vi "AudioTest.Discrete Swept-Sine Measurements (Finite).vi"() -> ()   [LabVIEW 2018]
doc: "Overview:\nThis VI demonstrates simultaneous frequency response, level, and distortion measurements using a discrete swept-sine technique. This example implements analog input and analog output with 'Finite Samples' sample mode which minimizes sensitivity to bandwidth issues that can cause run-time errors when performing continuous measurements. This VI also demonstrates how finite acquisitions can be read in a single large block or in a series of smaller reads.\n\nRequirements:\nLabVIEW Full Development System\nSound and Vibration Toolkit\n\nInstructions:\n1. Connect the DUT to the DSA device.\n2. Select the AO excitation channel, AI stimulus channel, and AI response channel.\n3. Run the VI.\n\nDetails:\nThis VI performs a swept sine measurement to obtain the root-mean-square (RMS) levels of the acquired stimulus and response, the frequency response of the device under test (DUT), and the harmonic distortion on the response channel. You specify the source and measurement parameters, and the swept sine VIs handle all the DAQ-specific controls required to perform the measurement. You have direct control over the source, input, averaging, and display parameters. You also specify the engineering units to use for the swept sine measurements.\n\nYou can view the time records of the acquired stimulus and response signals. From these graphs, you can see that the transition to the next test frequency always occurs at a zero crossing to minimize non-linear disturbances to the DUT. The RMS levels, frequency response, and harmonic distortion are shown on different tabs."
uses:
  <vilib>/sound2/lvsound2.llb/Sampling Mode.ctl
  <vilib>/sound2/lvsound2.llb/Sound Data Format.ctl
  <vilib>/Utility/error.llb/DialogType.ctl
  <vilib>/addons/_NISVFA/_Generation/Signal Generation/SV Signal/SV Signal.lvclass/SV Signal.ctl
  <vilib>/addons/_NISVFA/_Generation/Signal Generation/SV Discrete Sweep/SV Discrete Sweep.lvclass/SV Discrete Sweep.ctl
  <vilib>/addons/Sound and Vibration/svt_Level/SVL AC & DC Level (Time) (1 Ch).vi
  <vilib>/addons/_NISVFA/_Shared subVIs/Common/SV Append Data (N Ch) (DBL).vi
  <vilib>/addons/_NISVFA/_Generation/Signal Generation/SV Signal/Write Leading Synchronization Pulse Enable.vi
  <vilib>/addons/_NISVFA/_Generation/Signal Generation/SV Discrete Sweep/Read All Frequencies and Amplitudes.vi
  <vilib>/addons/_NISVFA/_Generation/Signal Generation/SV Discrete Sweep/Write All Frequencies and Amplitudes.vi
  <vilib>/addons/_NISVFA/_Shared subVIs/Common/svc_Get SV Channel Info.vi
  <vilib>/Analysis/baseanly.llb/Mean.vi
  <vilib>/Analysis/baseanly.llb/Mean (DBL).vi
  <vilib>/addons/_NISVFA/_Shared subVIs/Windowing/svfa_Scaled Time Domain Window (Array).vi
  <vilib>/addons/_NISVFA/_Generation/Signal Generation/SV Discrete Sweep/Read Frequencies and Amplitudes.vi
  <vilib>/Analysis/4window.llb/Force Window.vi
  <vilib>/Analysis/4window.llb/Force Window (DBL).vi
  <vilib>/Analysis/4window.llb/Exponential Window.vi
  <vilib>/Analysis/4window.llb/Exponential Window (DBL).vi
  <vilib>/addons/_NISVFA/_Generation/Signal Generation/SV Discrete Sweep/SV Discrete Sweep.lvclass
  C:/Program Files (x86)/National Instruments/LabVIEW 2018/vi.lib/addons/_NISVFA/_Generation/Signal Generation/SV Signal/SV Signal.lvclass
  C:/Program Files (x86)/National Instruments/LabVIEW 2018/vi.lib/addons/_NISVFA/_Generation/Signal Generation/SV Function/SV Function.lvclass
  <vilib>/addons/_NISVFA/_Generation/Signal Generation/SV Discrete Sweep/Configure Frequency Sweep at Constant Amplitude.vi
  <vilib>/addons/_NISVFA/_Generation/Signal Generation/SV Signal/Write Ramp Parameters.vi
  <vilib>/addons/_NISVFA/_Generation/Signal Generation/SV Signal/Write DC Offset.vi
  <vilib>/addons/_NISVFA/_Generation/Signal Generation/SV Signal/Write Measurement Duration.vi
  <vilib>/addons/_NISVFA/_Generation/Signal Generation/SV Function/Write Measurement Cycles.vi
  <vilib>/addons/_NISVFA/_Generation/Signal Generation/SV Signal/Write Pre-Measurement Settling Duration.vi
  <vilib>/addons/_NISVFA/_Generation/Signal Generation/SV Function/Write Pre-Measurement Settling Cycles.vi
  <vilib>/addons/_NISVFA/_Generation/Signal Generation/SV Signal/Write Sample Rate.vi
  <vilib>/sound2/lvsound2.llb/Sound Output Set Volume (Single).vi
  <vilib>/sound2/lvsound2.llb/Sound Output Write (DBL Single).vi
  <vilib>/sound2/lvsound2.llb/Sound Input Read (DBL).vi
  <vilib>/addons/_NISVFA/_Shared subVIs/Data Objects/Waveforms (DBL)/SV Read Next Measurement Data.vi
  <vilib>/addons/_NISVFA/_Shared subVIs/Common/svc_Get Window Info.vi
  <vilib>/addons/_NISVFA/_Shared subVIs/Common/svc_Unit Label to Engineering Units.vi
  <vilib>/addons/_NISVFA/_Shared subVIs/Common/svc_Engineering Units to Unit Label.vi
  <vilib>/addons/_NISVFA/_Spectrum Processing/subVIs/svfa_Spectrum Info Window to windowTd Type Def.vi
  <vilib>/Analysis/0measdsp.llb/Scaled Time Domain Window.vi
  <vilib>/Analysis/0measdsp.llb/Scaled Time Domain Window (DBL).vi
  <vilib>/Utility/error.llb/Error Cluster From Error Code.vi
  <vilib>/Analysis/baseanly.llb/Std Deviation and Variance.vi
  <vilib>/addons/_NISVFA/_Shared subVIs/Common/svc_Caller VI Returned in Error Source.vi
  <vilib>/addons/Sound and Vibration/svt_Single Tone Measurements/SVT Gain and Phase (Time).vi
  <vilib>/addons/Sound and Vibration/svt_Distortion/SVT THD and Harmonic Components (Frequency) (1 Ch).vi
  <vilib>/addons/_NISVFA/_Generation/Signal Generation/SV Signal/SV Signal.lvclass
  <vilib>/addons/_NISVFA/_Shared subVIs/Data Objects/Waveforms (DBL)/Waveforms (N Ch).lvclass
  <vilib>/addons/Sound and Vibration/svt_Distortion/SoundVib_Distortion.lvlib
  <vilib>/addons/Sound and Vibration/svt_Single Tone Measurements/SoundVib_SingleTone.lvlib
  Program Files (x86)/National Instruments/LabVIEW 2018/examples/Sound and Vibration/SoundVib_Audio Examples.lvlib
  C:/Program Files (x86)/National Instruments/LabVIEW 2018/vi.lib/addons/_NISVFA/_Generation/Signal Generation/SV Sinusoid/SV Sinusoid.lvclass
panel:
  in  "volume":dbl=40.0 format="%#_13g"
  in  "Play Cal Output":bool
  in  "Speaker Cal":path=path "C:/MTE/Utah Core Audio Test/Config/Speaker Calibration, PN XXX, SN YYY, v10-30-18.csv"
  out "Cal Speaker Out":waveform(dbl)(graph)
  out "Raw Mic":waveform(dbl)(graph)
  out "Mic dt":dbl
  out "Play dt":dbl
  out "Size Play":i32
  out "Size Mic":i32
  out "Data Cnt":i32
  out "Error":errorcluster
  out "error Mic":errorcluster
  out "error Spkr":errorcluster
  out "test time":u32
  in  "sweep settings":T1(tab)
  in  "device In":u32
  in  "device Out":u32=1
  in  "Samples/Sec":dbl=51200.0
  in  "Dur(s)":dbl=2.0 format="%.2p"
  out "CalcDur(s)":dbl=1.0 format="%.2p"
  in  "number of steps":i32=190 min=1
  in  "DC offset [V]":dbl format="%.2f"
  in  "amplitude [V]":dbl=1.0 format="%.2p"
  in  "frequency spacing":enum16{"Linear", "Logarithmic"}(ring)=enum."Logarithmic"
  in  "sweep range":cluster{"start":dbl, "stop":dbl}={"start"=20000.0, "stop"=100.0} {"stop" min=0.0 format="%.2f"; "start" min=0.0 format="%.2f"}
  in  "measurement":cluster{"time":dbl, "cycles":dbl}={"time"=0.001, "cycles"=10.0} {"cycles" min=5.0 max=1000.0 step=1.0; "time" min=0.0 max=5.0 step=0.0001 format="%.3f s"}
  in  "settling":cluster{"time":dbl, "cycles":dbl}={"time"=0.0, "cycles"=1.0} {"cycles" min=0.0 max=100.0 step=0.5; "time" min=0.0 max=5.0 step=0.0001 format="%.3f s"}
  in  "views":T2(tab)
  out "Response":waveform(dbl)[](graph)
  out "Stimulus":waveform(dbl)[](graph)
  out "RMS level (response)":cluster{"frequency":dbl[], "magnitude":dbl[]}(graph)
  out "RMS level (stimulus)":cluster{"frequency":dbl[], "magnitude":dbl[]}(graph)
  out "Phase":cluster{"frequency":dbl[], "magnitude":dbl[]}(graph)
  out "Magnitude":cluster{"frequency":dbl[], "magnitude":dbl[]}(graph)
  out "Harmonics":cluster{"f":dbl[], "H_i":dbl[]}[](graph)
  out "THD":cluster{"frequency":dbl[], "THD":dbl[]}(graph)
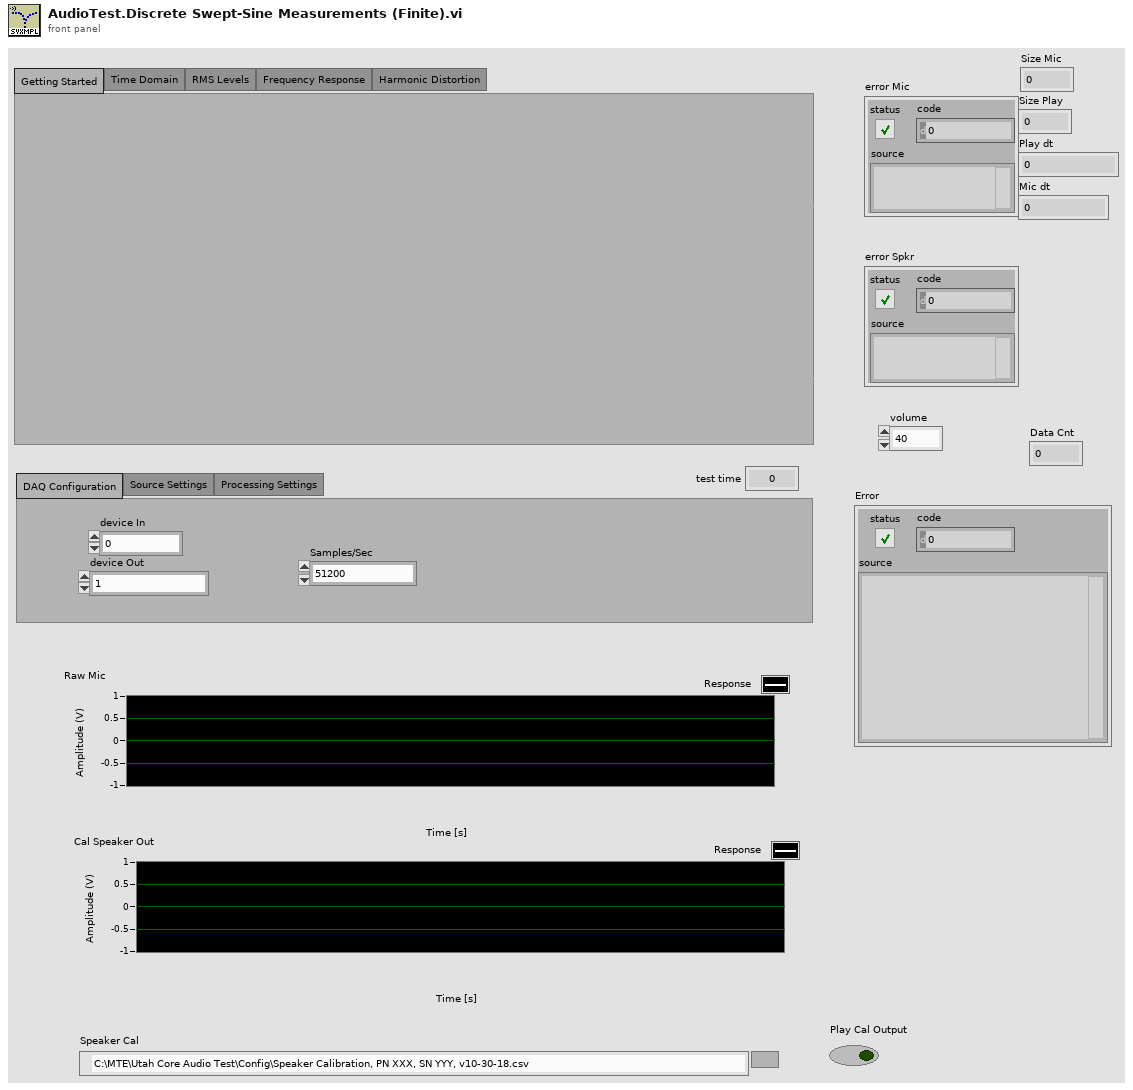
[diagram p1: front panel]
types:
  T1 = enum32{"DAQ Configuration", "Source Settings", "Processing Settings"}
  T2 = enum32{"Getting Started", "Time Domain", "RMS Levels", "Frequency Response", "Harmonic Distortion"}
  T3 = typedef "DialogType.ctl" = u16
  T4 = typedef "Sound Data Format.ctl" = cluster{"sample rate (S/s)":dbl, "number of channels":i32, "bits per sample":i32}
  T5 = typedef "Sampling Mode.ctl" = i32
  T6 = cluster{"profile":enum16{"Linear", "Half cosine"}, "durations [s]":cluster{"ramp-up":dbl, "transition":dbl, "ramp-down":dbl}}
  T7 = cluster{"frequency [Hz]":dbl, "amplitude [V]":dbl}[]
  T8 = typedef "Sound Output Task ID.ctl" = u32
  T9 = typedef "Sound Input Task ID.ctl" = u32
  T10 = cluster{"gain units":enum16{"dB", "linear ratio"}, "phase units":enum16{"deg", "rad"}, "detected tone stimulus amplitude units":enum16{"EU rms", "EU peak", "EU peak-peak"}, "detected tone response amplitude units":enum16{"EU rms", "EU peak", "EU peak-peak"}}
  T11 = cluster{"THD units":enum16{"dB", "linear ratio", "%"}, "harmonic component amplitude units":enum16{"EU rms", "EU peak", "EU peak-peak", "dB ref fund"}, "detected fundamental amplitude units":enum16{"EU rms", "EU peak", "EU peak-peak"}}
  T12 = typedef "svc_Spectrum Info.ctl" = cluster{"channel name":string, "description":string, "x-axis units":T13, "spectral info":cluster{"spectrum type":T14, "linear/dB":enum16{"linear", "dB"}, "window":u16, "window size":i32, "FFT size":i32}, "engineering units":T15, "custom label":string, "dB reference [EU]":dbl, "peak units":enum16{"rms", "peak", "peak-peak"}, "weighting filter":T16, "spectral density?":bool, "unit label":string, "spectrum skewed?":bool, "complimentary spectrum units":T17}
  T13 = typedef "svc_X-Axis Units.ctl" = u16
  T14 = typedef "svc_Spectrum Type.ctl" = enum16{"FFT Spectrum [complex]", "Amplitude [Magnitude]", "Power [Magnitude^2]", "Cross Spectrum [complex]", "Frequency Response [Complex]"}
  T15 = typedef "svc_Engineering Units Text Ring.ctl" = u16
  T16 = typedef "svc_Weighting Filter Text Ring.ctl" = u16
  T17 = typedef "svc_Complimentary Spectrum Units.ctl" = enum16{"none", "radians", "degrees", "cycles", "imaginary"}
  T18 = cluster{"complex spectrum response":cluster{"f0":dbl, "df":dbl, "complex spectrum":cdb[]}, "spectrum info":T12}
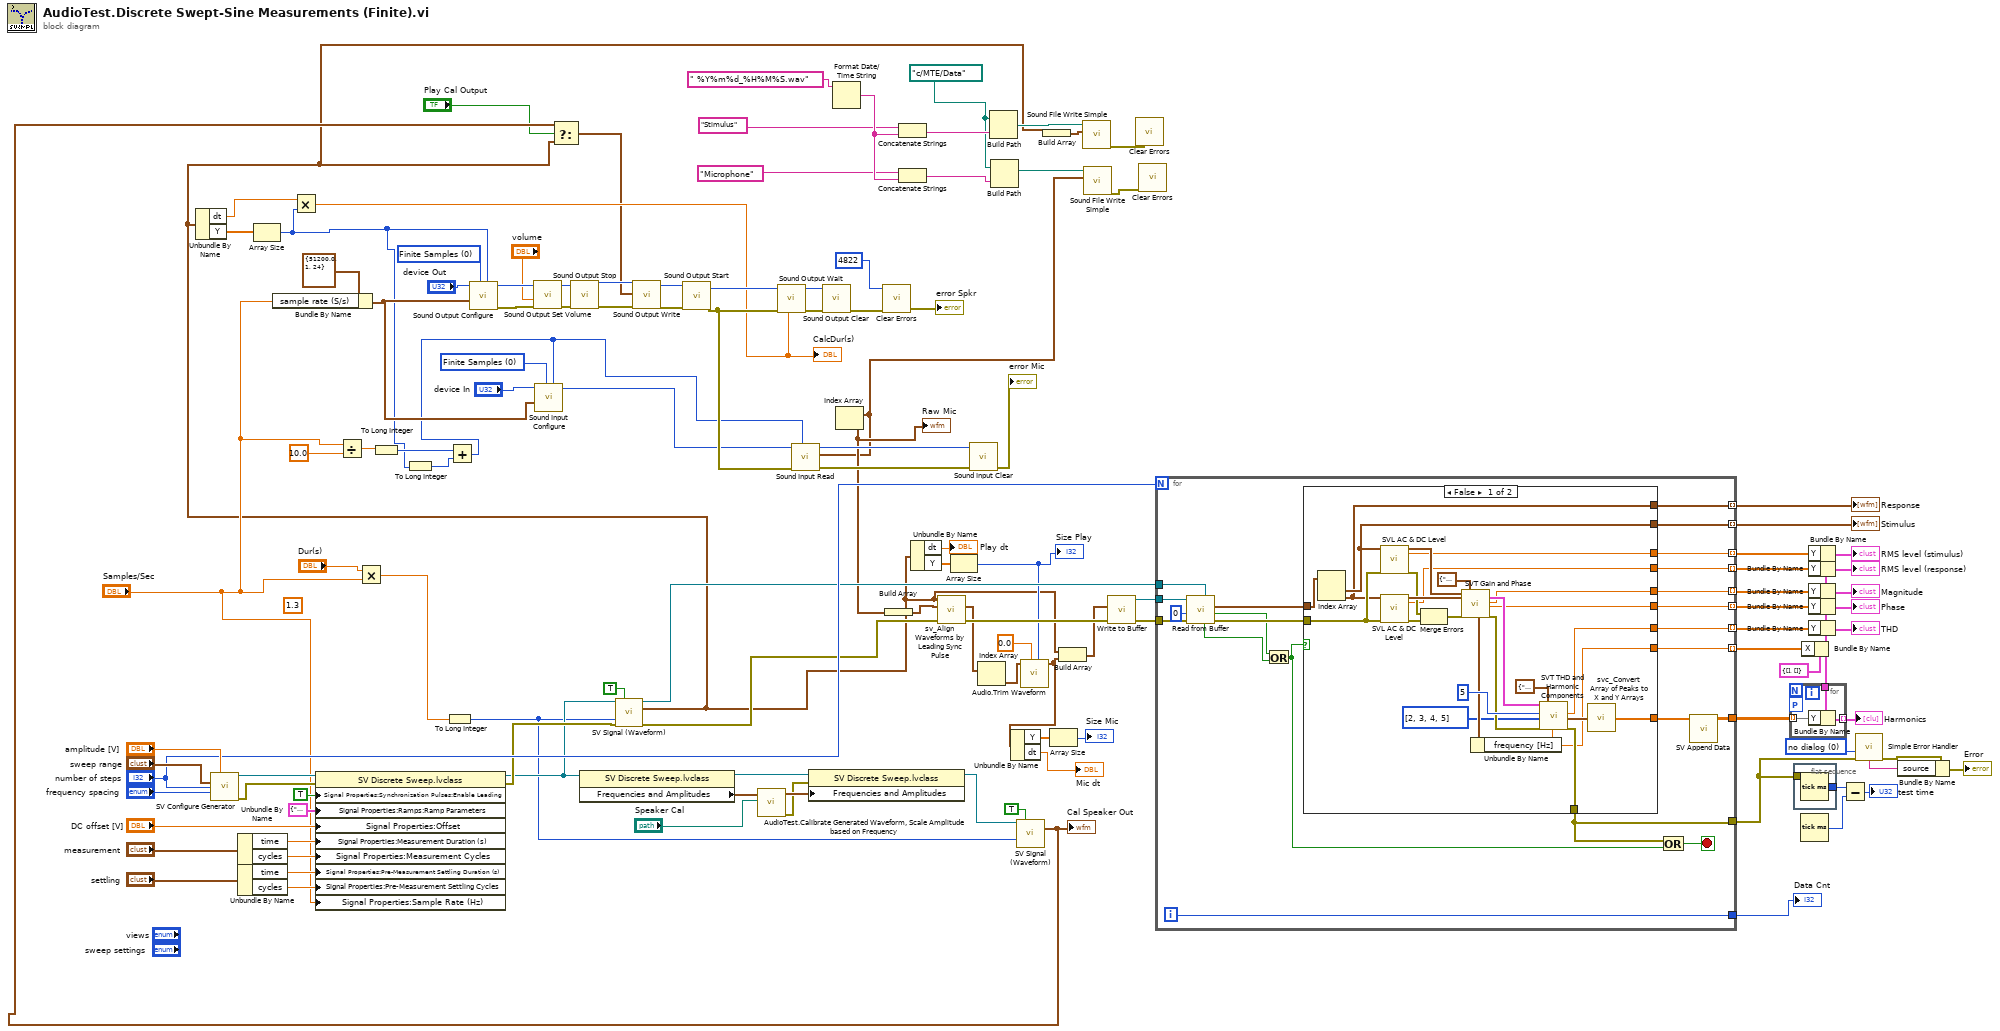
[diagram p0: block diagram]
diagram:
  w10 = path "c:/MTE/Data"
  w39 = T3 0 items=["no dialog", "OK message", "continue or stop message", "OK message + warnings", "continue/stop + warnings"] ("type of dialog (OK msg:1)")
  (unwired) 1.3 ("y")
  w76 = T5 0 items=["Finite Samples", "Continuous Samples"] ("sample mode")
  w78 = T5 0 items=["Finite Samples", "Continuous Samples"] ("sample mode")
  n1 = call-poly <vilib>:"SV Configure Generator.vi"("amplitude"="amplitude [V]", "frequency range [Hz]"="sweep range", "number of steps"="number of steps", "profile"="frequency spacing") -> ("signal configuration"=w125:refnum<class "SV Discrete Sweep.lvclass">, "error out"=w114:errorcluster)  [unwired: 10 in]
  n2 = Unbundle By Name("measurement") -> ("time"=w121:dbl, "cycles"=w120:dbl)
  n3 = Unbundle By Name("settling") -> ("time"=w123:dbl, "cycles"=w122:dbl)
  n4 = Bundle By Name(cluster=T4 {"sample rate (S/s)"=51200.0, "number of channels"=1, "bits per sample"=24} ("sound format"), "sample rate (S/s)"="Samples/Sec") -> (w70:T4)
  n5 = property class="SV Discrete Sweep.lvclass"(reference=w125, error in=w114, "Signal Properties:Synchronization Pulses:Enable Leading"=TRUE ("Synchronization Pulses:Enable Leading"), "Signal Properties:Ramps:Ramp Parameters"=T6 {"profile"=enum."Half cosine", "durations [s]"={"ramp-up"=0.01, "transition"=0.0, "ramp-down"=0.01}} ("Ramp Parameters"), "Signal Properties:Offset"="DC offset [V]", "Signal Properties:Measurement Duration (s)"=w121, "Signal Properties:Measurement Cycles"=w120, "Signal Properties:Pre-Measurement Settling Duration (s)"=w123, "Signal Properties:Pre-Measurement Settling Cycles"=w122, "Signal Properties:Sample Rate (Hz)"="Samples/Sec") -> (reference out=w26:refnum<class "SV Discrete Sweep.lvclass">, error out=w85:errorcluster)
  n6 = Divide(x="Samples/Sec", y=10.0) -> (x/y=w67:dbl)
  n7 = Multiply(x="Dur(s)", y="Samples/Sec") -> (x*y=w27:dbl)
  n8 = To Long Integer(number=w67) -> (32bit integer=w66:i32)
  n9 = To Long Integer(number=w27) -> (32bit integer=w20:i32)
  n10 = property class="SV Discrete Sweep.lvclass"(reference=w26) -> (reference out=w23:refnum<class "SV Discrete Sweep.lvclass">, "Frequencies and Amplitudes"=w25:T7)  [unwired: 1 in, 1 out]
  n11 = call-dynamic "SV Signal (Waveform).vi"("signal configuration"=w26, "reset"=TRUE, "samples"=w20, "error in (no error)"=w85) -> ("signal configuration"=w84:refnum<class "SV Discrete Sweep.lvclass">, "output waveform"=w6:waveform(dbl), "error out"=w83:errorcluster)  [unwired: 6 in, 3 out]
  n12 = Unbundle By Name(w6) -> ("dt"=w49:dbl, "Y"=w69:dbl[])
  n13 = Array Size(array=w69) -> (size(s)=w50:i32)
  n14 = Multiply(x=w49, y=w50) -> (x*y=w48:dbl)
  "CalcDur(s)" <- w48
  n15 = To Long Integer(number=w50) -> (32bit integer=w65:i32)
  n16 = Add(x=w66, y=w65) -> (x+y=w56:i32)
  n17 = call <vilib>:"Sound Output Configure.vi"("number of samples/ch"=w50, "sample mode"=w78, "sound format"=w70, "device ID"="device Out") -> ("error out"=w82:errorcluster, "task ID"=w81:T8)  [unwired: 6 in]
  n18 = call-poly <vilib>:"Sound Output Set Volume.vi"("error in (no error)"=w82, "volume"="volume", "task ID"=w81) -> ("error out"=w74:errorcluster, "task ID out"=w75:T8)  [unwired: 7 in]
  n19 = call <vilib>:"Sound Input Configure.vi"("number of samples/ch"=w56, "sample mode"=w76, "sound format"=w70, "device ID"="device In") -> ("task ID"=w55:T9)  [unwired: 6 in, 1 out]
  n20 = call <vilib>:"Sound Output Stop.vi"("error in (no error)"=w74, "task ID"=w75) -> ("error out"=w72:errorcluster, "task ID out"=w73:T8)  [unwired: 8 in]
  n21 = call "AudioTest.Calibrate Generated Waveform, Scale Amplitude based on Frequency.vi"("Calibration File"="Speaker Cal", "Frequencies and Amplitudes"=w25) -> ("error out"=w1:errorcluster, "Frequencies and Amplitudes Out"=w24:T7)  [unwired: 8 in]
  n22 = property class="SV Discrete Sweep.lvclass"(reference=w23, error in=w1, "Frequencies and Amplitudes"=w24) -> (reference out=w21:refnum<class "SV Discrete Sweep.lvclass">)  [unwired: 1 out]
  n23 = Format Date/Time String(time format string (%c)=" %Y%m%d_%H%M%S.wav") -> (date/time string=w15:string)  [unwired: 2 in]
  n24 = Concatenate Strings("Stimulus", w15) -> (w11:string)
  n25 = Concatenate Strings("Microphone", w15) -> (w9:string)
  n26 = Unbundle By Name(w6) -> ("dt"=→"Play dt":dbl, "Y"=w40:dbl[])
  n27 = Array Size(array=w40) -> (size(s)=w32:i32)
  "Size Play" <- w32
  n28 = Build Path(base path=w10, name or relative path=w11) -> (appended path=w12:path)
  n29 = Build Path(base path=w10, name or relative path=w9) -> (appended path=w8:path)
  n30 = call-dynamic "SV Signal (Waveform).vi"("signal configuration"=w21, "reset"=TRUE, "samples"=w20) -> ("output waveform"=w18:waveform(dbl))  [unwired: 7 in, 5 out]
  "Cal Speaker Out" <- w18
  n31 = Select(t=w18, s="Play Cal Output", f=w6) -> (s? t:f=w7:waveform(dbl))
  n32 = call-poly <vilib>:"Sound Output Write.vi"("error in (no error)"=w72, "data"=w7, "task ID"=w73) -> ("error out"=w57:errorcluster, "task ID out"=w58:T8)  [unwired: 7 in]
  n33 = call <vilib>:"Sound Output Start.vi"("error in (no error)"=w57, "task ID"=w58) -> ("error out"=w61:errorcluster, "task ID out"=w62:T8)  [unwired: 8 in]
  n34 = call <vilib>:"Sound Output Wait.vi"("timeout (sec)"=w48, "error in (no error)"=w61, "task ID"=w62) -> ("error out"=w64:errorcluster, "task ID out"=w63:T8)  [unwired: 7 in]
  n35 = call-poly <vilib>:"Sound Input Read.vi"("number of samples/ch"=w56, "error in (no error)"=w61, "task ID"=w55) -> ("error out"=w53:errorcluster, "data"=w4:waveform(dbl)[], "task ID out"=w54:T9)  [unwired: 6 in]
  n36 = call <vilib>:"Sound Output Clear.vi"("error in (no error)"=w64, "task ID"=w63) -> ("error out"=w60:errorcluster)  [unwired: 9 in]
  n37 = Index Array(array=w4) -> (element=w29:waveform(dbl))  [unwired: 1 in]
  "Raw Mic" <- w29
  n38 = call <vilib>:"Clear Errors.vi"("error in (no error)"=w60, "specific error code to clear (0: all)"=4822) -> ("error out"=→"error Spkr":errorcluster)  [unwired: 4 in, 1 out]
  n39 = Build Array(w29) -> (w45:waveform(dbl)[])
  n40 = call "sv_Align Waveforms by Leading Sync Pulse.vi"("error in (no error)"=w83, "response signals"=w45, "alignment reference signal"=w6) -> ("error out"=w87:errorcluster, "aligned signals"=w43:waveform(dbl)[])  [unwired: 4 in, 3 out]
  n41 = call <vilib>:"Sound Input Clear.vi"("error in (no error)"=w53, "task ID"=w54) -> ("error out"=→"error Mic":errorcluster)  [unwired: 9 in]
  n42 = Index Array(array=w43) -> (element=w44:waveform(dbl))  [unwired: 1 in]
  n43 = call "Audio.Trim Waveform.vi"("Len"=w32, "Max Delay"=0.0, "Data In"=w44) -> ("Data Out"=w34:waveform(dbl))  [unwired: 8 in]
  n44 = Unbundle By Name(w34) -> ("Y"=w35:dbl[], "dt"=→"Mic dt":dbl)
  n45 = Build Array(w6) -> (w5:waveform(dbl)[])
  n46 = Array Size(array=w35) -> (size(s)=→"Size Mic":i32)
  n47 = Build Array(w6, w34) -> (w42:waveform(dbl)[])
  n48 = call <vilib>:"Sound File Write Simple.vi"("data"=w5, "path"=w12) -> ("error out"=w3:errorcluster)  [unwired: 8 in, 1 out]
  n49 = call <vilib>:"Sound File Write Simple.vi"("data"=w4, "path"=w8) -> ("error out"=w2:errorcluster)  [unwired: 8 in, 1 out]
  n50 = call <vilib>:"Write to Buffer.vi"("error in (no error)"=w87, "waveforms"=w42) -> ("error out"=w88:errorcluster, "buffer out"=w89:refnum<data-value>)  [unwired: 7 in, 1 out]
  n51 = call <vilib>:"Clear Errors.vi"("error in (no error)"=w3) -> ()  [unwired: 5 in, 2 out]
  n52 = call <vilib>:"Clear Errors.vi"("error in (no error)"=w2) -> ()  [unwired: 5 in, 2 out]
  n53 = for {
    N: "number of steps" -> [_]
    tunnel: w89 -> [w145]
    tunnel: w84 -> [w144]
    tunnel: w88 -> [w143]
    tunnel: [w131] -> w94
    tunnel: [w140] -> w106 mode=indexing
    tunnel: [w139] -> w105 mode=indexing
    tunnel: [w138] -> w104 mode=indexing
    tunnel: [w137] -> w103 mode=indexing
    tunnel: [w136] -> w102 mode=indexing
    tunnel: [w127] -> w98 mode=indexing
    tunnel: [w134] -> w97
    tunnel: [w133] -> w96 mode=indexing
    tunnel: [w132] -> w95 mode=indexing
    tunnel: [w128] -> w28
    i -> [w128]
    stop <- w141 stop-if-true
    n54 = call-poly <vilib>:"Read from Buffer.vi"("test signal configuration"=w144, "error in (no error)"=w143, "timeout (1000 ms)"=0, "buffer"=w145) -> ("error out"=w147:errorcluster, "end of buffer"=w130:bool, "waveforms subset"=w142:waveform(dbl)[], "done"=w129:bool)  [unwired: 3 in, 1 out]
    n55 = Or(x=w130, y=w129) -> (x .or. y?=w126:bool)
    n56 = case shown="False" w126 {
      tunnel: w147 -> [w172 _]
      tunnel: w142 -> [w171 _]
      tunnel: [w157 _] -> w140
      tunnel: [w156 _] -> w139
      tunnel: [w155 _] -> w138
      tunnel: [w154 _] -> w137
      tunnel: [w153 _] -> w136
      tunnel: [w152 _] -> w135
      tunnel: [w151 _] -> w133
      tunnel: [w150 _] -> w132
      tunnel: [w149 _] -> w131
      tunnel: [w148 _] -> w127
      frame False {
        n57 = Index Array(array=w171) -> (element #1=w151:waveform(dbl), element #2=w150:waveform(dbl))  [unwired: 2 in]
        n58 = call-poly <vilib>:"SVL AC & DC Level.vi"("scaled signal [EU]"=w151, "error in (no error)"=w172) -> ("AC signal [EU]"=w165:waveform(dbl), "AC level [EU rms]"=w157:dbl, "error out"=w162:errorcluster)  [unwired: 12 in, 3 out]
        n59 = call-poly <vilib>:"SVL AC & DC Level.vi"("scaled signal [EU]"=w150, "error in (no error)"=w172) -> ("AC signal [EU]"=w164:waveform(dbl), "AC level [EU rms]"=w156:dbl, "error out"=w161:errorcluster)  [unwired: 12 in, 3 out]
        n60 = Merge Errors(w162, w161) -> (w160:errorcluster)
        n61 = call-poly <vilib>:"SVT Gain and Phase.vi"("stimulus signal X [EUx]"=w165, "response signal Y [EUy]"=w164, "error in (no error)"=w160, "desired units"=T10 {"gain units"=enum."dB", "phase units"=enum."deg", "detected tone stimulus amplitude units"=enum."EU rms", "detected tone response amplitude units"=enum."EU rms"}) -> ("detected tone response"=w159:cluster{"frequency [Hz]":dbl, "amplitude":dbl}, "complex spectrum\nresponse Y"=w166:T18, "gain"=w155:dbl, "phase lag"=w154:dbl, "error out"=w163:errorcluster)  [unwired: 8 in, 3 out]
        n62 = Unbundle By Name(w159) -> ("frequency [Hz]"=w148:dbl)
        n63 = call-poly <vilib>:"SVT THD and Harmonic Components.vi"("complex spectrum"=w166, "maximum harmonic"=5, "harmonics to visualize"=i32[] [2, 3, 4, 5], "error in (no error)"=w163, "desired units"=T11 {"THD units"=enum."dB", "harmonic component amplitude units"=enum."dB ref fund", "detected fundamental amplitude units"=enum."EU peak"}, "expected fundamental frequency [Hz]"=w148) -> ("THD"=w153:dbl, "harmonic components"=w167:cluster{"frequency [Hz]":dbl, "amplitude":dbl}[], "error out"=w149:errorcluster)  [unwired: 6 in, 5 out]
        n64 = call <vilib>:"svc_Convert Array of Peaks to X and Y Arrays.vi"("peaks"=w167) -> ("Y"=w152:dbl[])  [unwired: 3 in, 1 out]
      }
      frame True {
      }
    }
    n65 = Compound Arithmetic op=OR(w131, w126) -> (w141:bool)
    n66 = call-poly <vilib>:"SV Append Data.vi"("data in"=w135) -> ("appended data"=w134:dbl[][])  [unwired: 10 in]
  }
  "Stimulus" <- w96
  "Response" <- w95
  "Data Cnt" <- w28
  n67 = flat-sequence {
    tunnel: w94 -> [_]
    tunnel: [w173] -> w93
    frame #0 {
      n68 = Tick Count (ms)() -> (millisecond timer value=w173:u32)
    }
  }
  n69 = Tick Count (ms)() -> (millisecond timer value=w91:u32)
  n70 = Bundle By Name(cluster=cluster{"X":dbl[], "Y":dbl[]} {"X"=[], "Y"=[]} ("THD vs Amplitude"), "X"=w98) -> (w99:cluster{"X":dbl[], "Y":dbl[]})
  n71 = for {
    tunnel: [w176] -> w101 mode=indexing
    tunnel: w99 -> [w175]
    workers-P: _ -> [_]
    tunnel: w97 -> [w174] mode=indexing
    n72 = Bundle By Name(cluster=w175, "Y"=w174) -> (w176:cluster{"X":dbl[], "Y":dbl[]})
  }
  "Harmonics" <- w101
  n73 = Bundle By Name(cluster=w99, "Y"=w106) -> (→"RMS level (stimulus)":cluster{"X":dbl[], "Y":dbl[]})
  n74 = Bundle By Name(cluster=w99, "Y"=w105) -> (→"RMS level (response)":cluster{"X":dbl[], "Y":dbl[]})
  n75 = Bundle By Name(cluster=w99, "Y"=w104) -> (→"Magnitude":cluster{"X":dbl[], "Y":dbl[]})
  n76 = Bundle By Name(cluster=w99, "Y"=w103) -> (→"Phase":cluster{"X":dbl[], "Y":dbl[]})
  n77 = Bundle By Name(cluster=w99, "Y"=w102) -> (→"THD":cluster{"X":dbl[], "Y":dbl[]})
  n78 = Subtract(x=w93, y=w91) -> (x-y=→"test time":u32)
  n79 = call <vilib>:"Simple Error Handler.vi"("type of dialog (OK msg:1)"=w39, "error in (no error)"=w94) -> ("error out"=w38:errorcluster, "message"=w37:string)  [unwired: 3 in, 3 out]
  n80 = Bundle By Name(cluster=w38, "source"=w37) -> (→"Error":errorcluster)
